vi "FindWidth.vi"(6 "theta":dbl=0.3 format="%#_13g", 7 "Center":dbl[](array[numeric]), 8 "Array in":i32[][](array[numeric])) -> (2 "height":dbl, 3 "width":dbl)   [LabVIEW 2017]
uses:
  <vilib>/Analysis/coordinate.llb/2D Cartesian Coordinate Shift (Array).vi
  <vilib>/Analysis/coordinate.llb/2D Cartesian Coordinate Rotation (Array).vi
  <vilib>/Analysis/NI_AALPro.lvlib
panel:
  out "appended array":dbl[][](array[numeric])
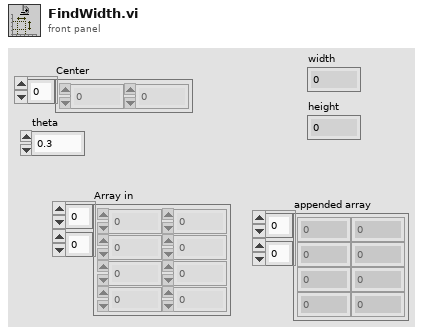
[diagram p1: front panel]
types:
  T1 = cluster{"Real Matrix Element":dbl, "Real Matrix Element":dbl}
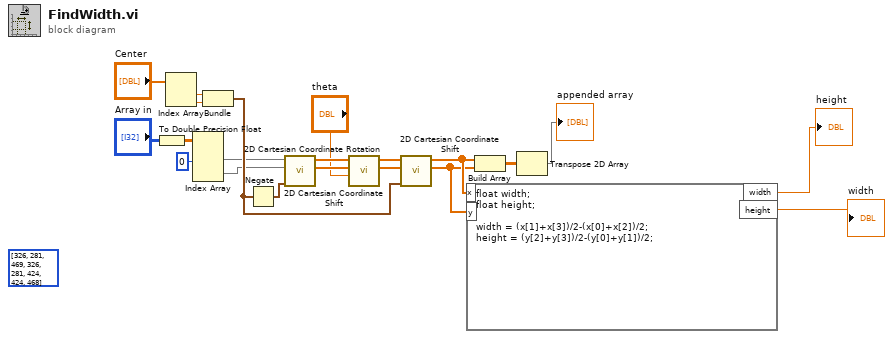
[diagram p0: block diagram]
diagram:
  (unwired) i32[][] [[326, 281], [469, 326], [281, 424], [424, 468]] ("Array in")
  n1 = To Double Precision Float(number="Array in") -> (double precision float=w9:dbl[][])
  n2 = Index Array(array="Center") -> (element #1=w14:dbl, element #2=w15:dbl)  [unwired: 2 in]
  n3 = Index Array(array=w9, index (col) #1=0 ("disabled index (col)")) -> (element #1=w12:dbl[], element #2=w13:dbl[])  [unwired: 3 in]
  n4 = Bundle("Real Matrix Element"=w14, "Real Matrix Element"=w15) -> (w20:T1)  [unwired: 1 in]
  n5 = Negate(x=w20) -> (-x=w21:T1)
  n6 = call-poly <vilib>:"2D Cartesian Coordinate Shift.vi"("shift"=w21, "Y"=w13, "X"=w12) -> ("Y Out"=w17:dbl[], "X Out"=w16:dbl[])  [unwired: 6 in, 1 out]
  n7 = call-poly <vilib>:"2D Cartesian Coordinate Rotation.vi"("theta"="theta", "Y"=w17, "X"=w16) -> ("Y Out"=w19:dbl[], "X Out"=w18:dbl[])  [unwired: 6 in, 1 out]
  n8 = call-poly <vilib>:"2D Cartesian Coordinate Shift.vi"("shift"=w20, "Y"=w19, "X"=w18) -> ("Y Out"=w3:dbl[], "X Out"=w4:dbl[])  [unwired: 6 in, 1 out]
  n9 = formula code="float width;\nfloat height;\n\nwidth = (x[1]+x[3])/2-(x[0]+x[2])/2;\nheight = (y[2]+y[3])/2-(y[0]+y[1])/2;"("x"=w4, "y"=w3) -> ("width"=→"height":dbl, "height"=→"width":dbl)
  n10 = Build Array(w4, w3) -> (w7:dbl[][])
  n11 = Transpose 2D Array(2D array=w7) -> (transposed array=→"appended array":dbl[][])
